vi "Lookup Control Type.vi"(10 "error in (no error)":errorcluster, 11 "Control Type":string) -> (2 "error out":errorcluster, 3 "ValveControl":refnum<class "DigitalControl.lvclass">)   [LabVIEW 2020, in "VolatusControl.lvlib" / "DigitalControlModule.lvclass"]
uses:
  DigitalControlModule.lvclass
  DigitalControlModule.lvclass/DigitalControlModule.ctl
  DigitalControl/DigitalControl.lvclass
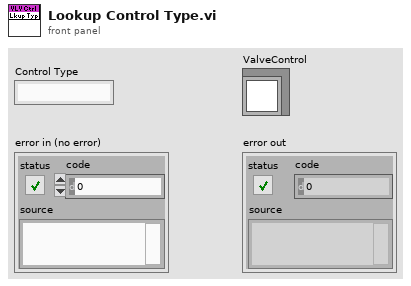
[diagram p1: front panel]
types:
  T1 = map{string, refnum<class "DigitalControl.lvclass">}
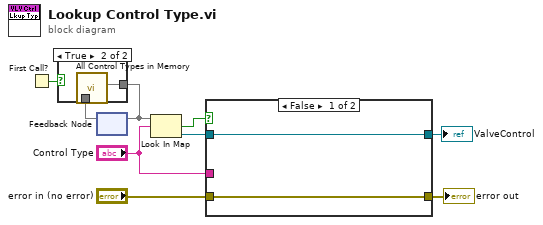
[diagram p0: block diagram]
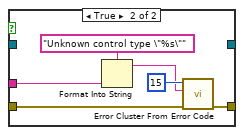
[diagram p2: hidden frame]
diagram:
  n1 = First Call?() -> (First Call?: T/F=w9:bool)
  n2 = feedback #1() -> (w8:T1)  [unwired: 1 in]
  n3 = case shown="True" w9 {
    tunnel: [w10 w11] -> w7
    tunnel: w8 -> [w10 _]
    frame False {
    }
    frame True {
      n4 = call "All Control Types in Memory.vi"() -> ("Control Types"=w11:T1)  [unwired: 11 in]
    }
  }
  n5 = feedback-in #1(w7) -> ()
  n6 = Look In Map(map=w7, key="Control Type") -> (key not found?=w6:bool, value=w5:refnum<class "DigitalControl.lvclass">)  [unwired: 1 in]
  n7 = case shown="False" w6 {
    tunnel: w5 -> [w13 _]
    tunnel: [w13 _] -> w4
    tunnel: "error in (no error)" -> [w12 w19]
    tunnel: [w12 w18] -> w2
    tunnel: "Control Type" -> [_ w14]
    frame False {
    }
    frame True {
      n8 = Format Into String(format string="Unknown control type \"%s\"", w14) -> (resulting string=w15:string)  [unwired: 2 in, 1 out]
      n9 = call <vilib>:"Error Cluster From Error Code.vi"("error in (no error)"=w19, "error message (\"\")"=w15, "error code (0)"=15) -> ("error out"=w18:errorcluster)  [unwired: 6 in]
    }
  }
  "ValveControl" <- w4
  "error out" <- w2
